vi "Burn-In Testing_v2.vi"() -> ()   [LabVIEW 2012]
uses:
  Controls/UserInput.ctl
  Controls/Instr_Param.ctl
  Controls/USB4000_Data.ctl
  Controls/MapPOS.ctl
  Controls/Waferimage.ctl
  Controls/MeasureControl.ctl
  Controls/TestArea.ctl
  Controls/TestData.ctl
  Controls/WaferTable.ctl
  Controls/Config.ctl
  Controls/AppPaths.ctl
  Controls/PathTraveler.ctl
  Controls/PathTypes.ctl
  Classes/EpiWrapper.lvclass
  TestData/Command.ctl
  Controls/Command_Enum.ctl
  Controls/Exit.vi
panel:
  in  "AppPaths":T1={"DataDir"={"Enum"=enum."DataDir", "FileName"="", "Exists?"=FALSE, "Path"=path ""}, "OmniDriver"={"Enum"=enum."OmniDriver", "FileName"="OmniDriver32.dll", "Exists?"=FALSE, "Path"=path ""}, "OmniDriverCommon"={"Enum"=enum."OmniDriver_Common", "FileName"="common32.dll", "Exists?"=FALSE, "Path"=path ""}, "Configuration"={"Enum"=enum."Configuration", "FileName"="TestConfiguration.cfg", "Exists?"=FALSE, "Path"=path ""}, "WaferImage"={"Enum"=enum."WaferImage", "FileName"="EPI_Wafer_Labels.jpg", "Exists?"=FALSE, "Path"=path ""}}
  in  "Configuration":T4={"IntTime"=100, "Samples"=3, "PowerMin"=300.0, "KneeMin"=-20.0, "KneeMax"=20.0, "BackgroundWl"=275.0} {"BackgroundWl" min=220.0 max=320.0; "IntTime" min=1 max=100000; "PowerMin" min=0.0 max=10000.0; "KneeMin" min=-40.0 max=0.0; "KneeMax" min=0.0 max=40.0; "Samples" min=1 max=10}
  out "Output For Excel":string
  in  "Integration Time(ms)\nMin=10ms":i32=10 min=10 max=100000
  out "Status":bool
  in  "Wafer Data,20mA":T5
  in  "MeasureControl":T6 {"TestData"."50mA Data"."Current,mA" format="%_6g"; "TestData"."50mA Data"."WL" format="%_6g"; "TestData"."50mA Data"."Voltage" format="%_6g"; "TestData"."50mA Data"."Power" format="%_6g"; "TestData"."20mA Data"."Reverse" format="%#_3g"; "TestData"."20mA Data"."Current,mA" format="%_6g"; "TestData"."20mA Data"."Knee Current" format="%#_3g"; "TestData"."20mA Data"."WL" format="%_6g"; "TestData"."20mA Data"."Voltage" format="%_6g"; "TestData"."20mA Data"."Power" format="%_5g"}
  out "Wafer":T9
  in  "MapPOS":T10={"Top"={"left"=208, "top"=106, "right"=218, "bottom"=116}, "CenterC"={"left"=217, "top"=189, "right"=228, "bottom"=200}, "CenterB"={"left"=217, "top"=208, "right"=228, "bottom"=219}, "CenterA"={"left"=199, "top"=208, "right"=209, "bottom"=219}, "Left"={"left"=103, "top"=199, "right"=114, "bottom"=209}, "Right"={"left"=314, "top"=199, "right"=325, "bottom"=209}}
  in  "INSTR_PARAM":T11
  in  "Stop":bool
  in  "Input":T13={"Wafer ID"="", "Test"="Initial", "New"=FALSE, "Save"=FALSE, "Load"=FALSE, "Cancel"=FALSE}
  # "Current Result"
  # "Measure Control"
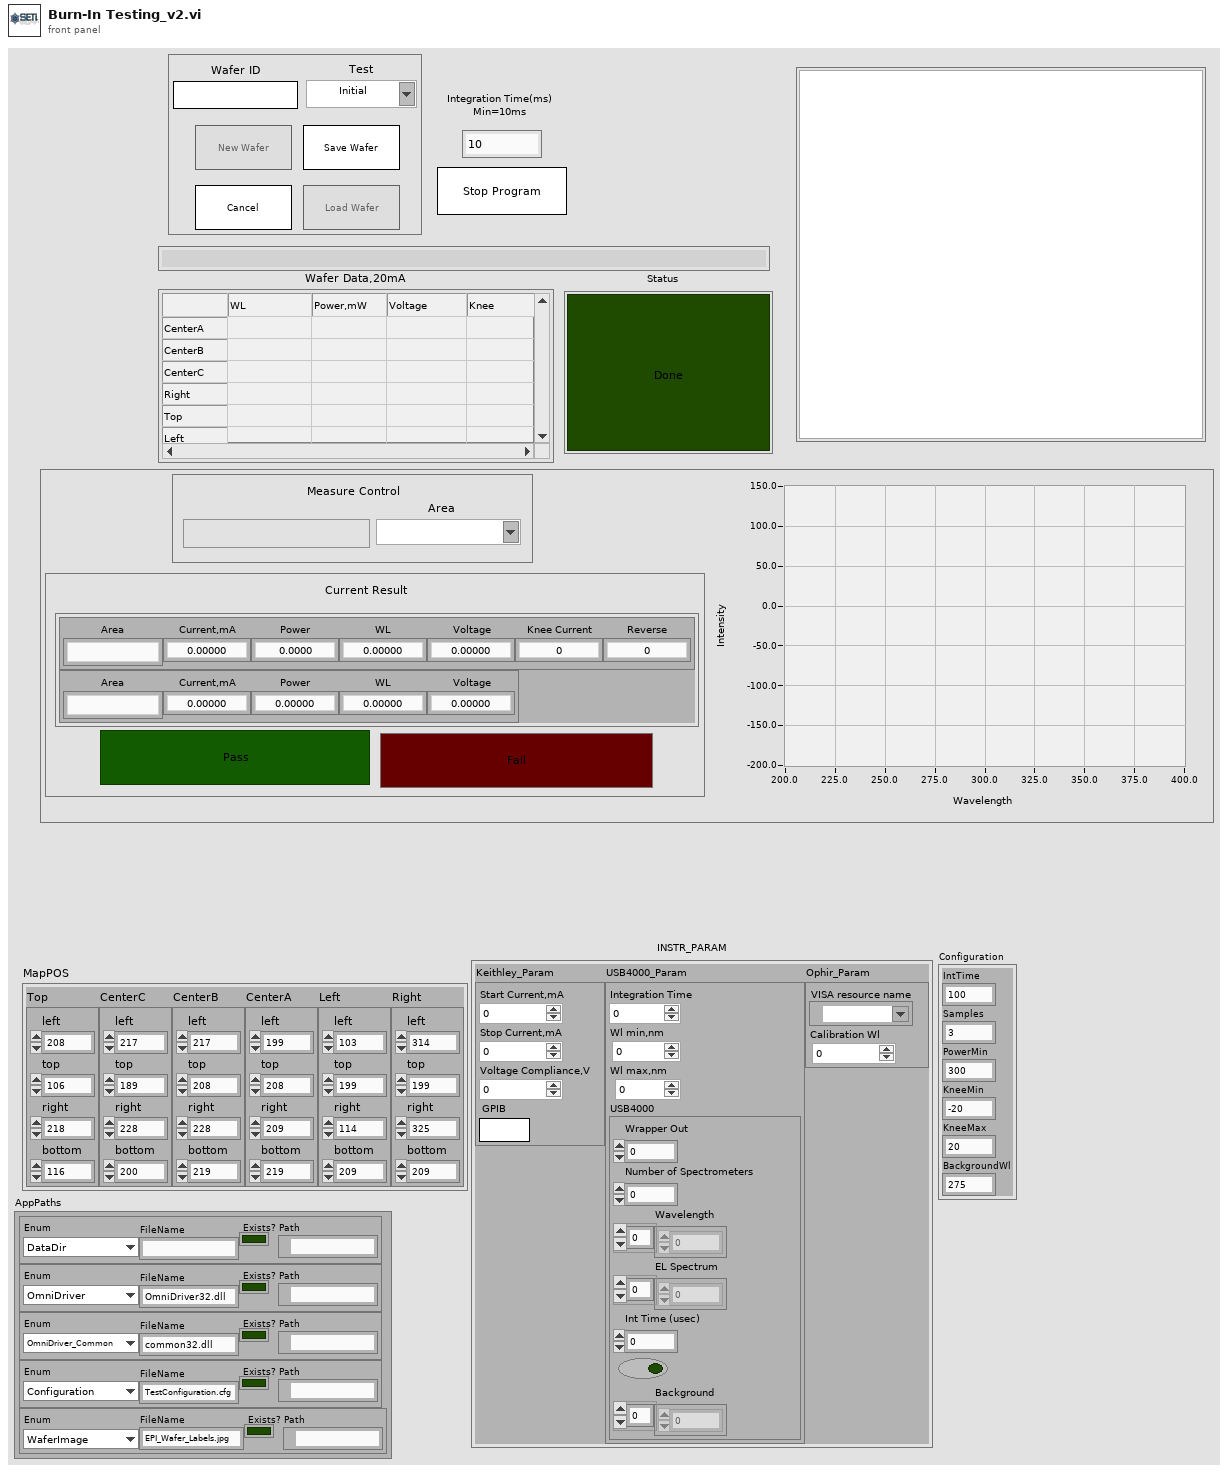
[diagram p1: front panel]
types:
  T1 = typedef "AppPaths.ctl" = cluster{"DataDir":T2, "OmniDriver":T2, "OmniDriverCommon":T2, "Configuration":T2, "WaferImage":T2}
  T2 = typedef "PathTraveler.ctl" = cluster{"Enum":T3, "FileName":string, "Exists?":bool, "Path":path}
  T3 = typedef "PathTypes.ctl" = enum16{"DataDir", "OmniDriver", "OmniDriver_Common", "Configuration", "WaferImage"}
  T4 = typedef "Config.ctl" = cluster{"IntTime":i32, "Samples":i32, "PowerMin":dbl, "KneeMin":dbl, "KneeMax":dbl, "BackgroundWl":dbl}
  T5 = typedef "WaferTable.ctl" = string[][]
  T6 = typedef "MeasureControl.ctl" = cluster{"Pass":bool, "Fail":bool, "Measure":bool, "Area":T7, "TestData":T8, "Graph":cluster{"Y":dbl[], "Y":dbl[]}[]}
  T7 = typedef "TestArea.ctl" = string
  T8 = typedef "TestData.ctl" = cluster{"20mA Data":cluster{"Area":string, "Current,mA":dbl, "Power":dbl, "WL":dbl, "Voltage":dbl, "Knee Current":dbl, "Reverse":dbl}, "50mA Data":cluster{"Area":string, "Current,mA":dbl, "Power":dbl, "WL":dbl, "Voltage":dbl}}
  T9 = typedef "Waferimage.ctl" = picture
  T10 = typedef "MapPOS.ctl" = cluster{"Top":cluster{"left":i16, "top":i16, "right":i16, "bottom":i16}, "CenterC":cluster{"left":i16, "top":i16, "right":i16, "bottom":i16}, "CenterB":cluster{"left":i16, "top":i16, "right":i16, "bottom":i16}, "CenterA":cluster{"left":i16, "top":i16, "right":i16, "bottom":i16}, "Left":cluster{"left":i16, "top":i16, "right":i16, "bottom":i16}, "Right":cluster{"left":i16, "top":i16, "right":i16, "bottom":i16}}
  T11 = typedef "Instr_Param.ctl" = cluster{"Keithley_Param":cluster{"Start Current,mA":dbl, "Stop Current,mA":dbl, "Voltage Compliance,V":dbl, "GPIB":string}, "USB4000_Param":cluster{"Integration Time":i32, "Wl min,nm":dbl, "Wl max,nm":dbl, "USB4000":T12}, "Ophir_Param":cluster{"VISA resource name":refnum<visa-resource-name>, "Calibration Wl":dbl}}
  T12 = typedef "USB4000_Data.ctl" = cluster{"Wrapper Out":u32, "Number of Spectrometers":i32, "Wavelength":dbl[], "EL Spectrum":dbl[], "Int Time (usec)":i32, bool, "Background":dbl[]}
  T13 = typedef "UserInput.ctl" = cluster{"Wafer ID":string, "Test":string, "New":bool, "Save":bool, "Load":bool, "Cancel":bool}
  T14 = typedef "Command.ctl" = cluster{"Command":T15, "Data":variant, "type":variant}
  T15 = typedef "Command_Enum.ctl" = enum16{"SPECTRUMCAPTURE", "RESETCONFIG", "OPENCONFIG", "RESET", "INIT", "LOAD", "MEASURE", "NEW", "SAVE", "UPDATE_INT", "SWAP_MODE", "UPDATE_ACQ", "EXIT", "CANCEL"}
  T16 = enum8{"Enabled", "Disabled", "Disabled and Grayed Out"}
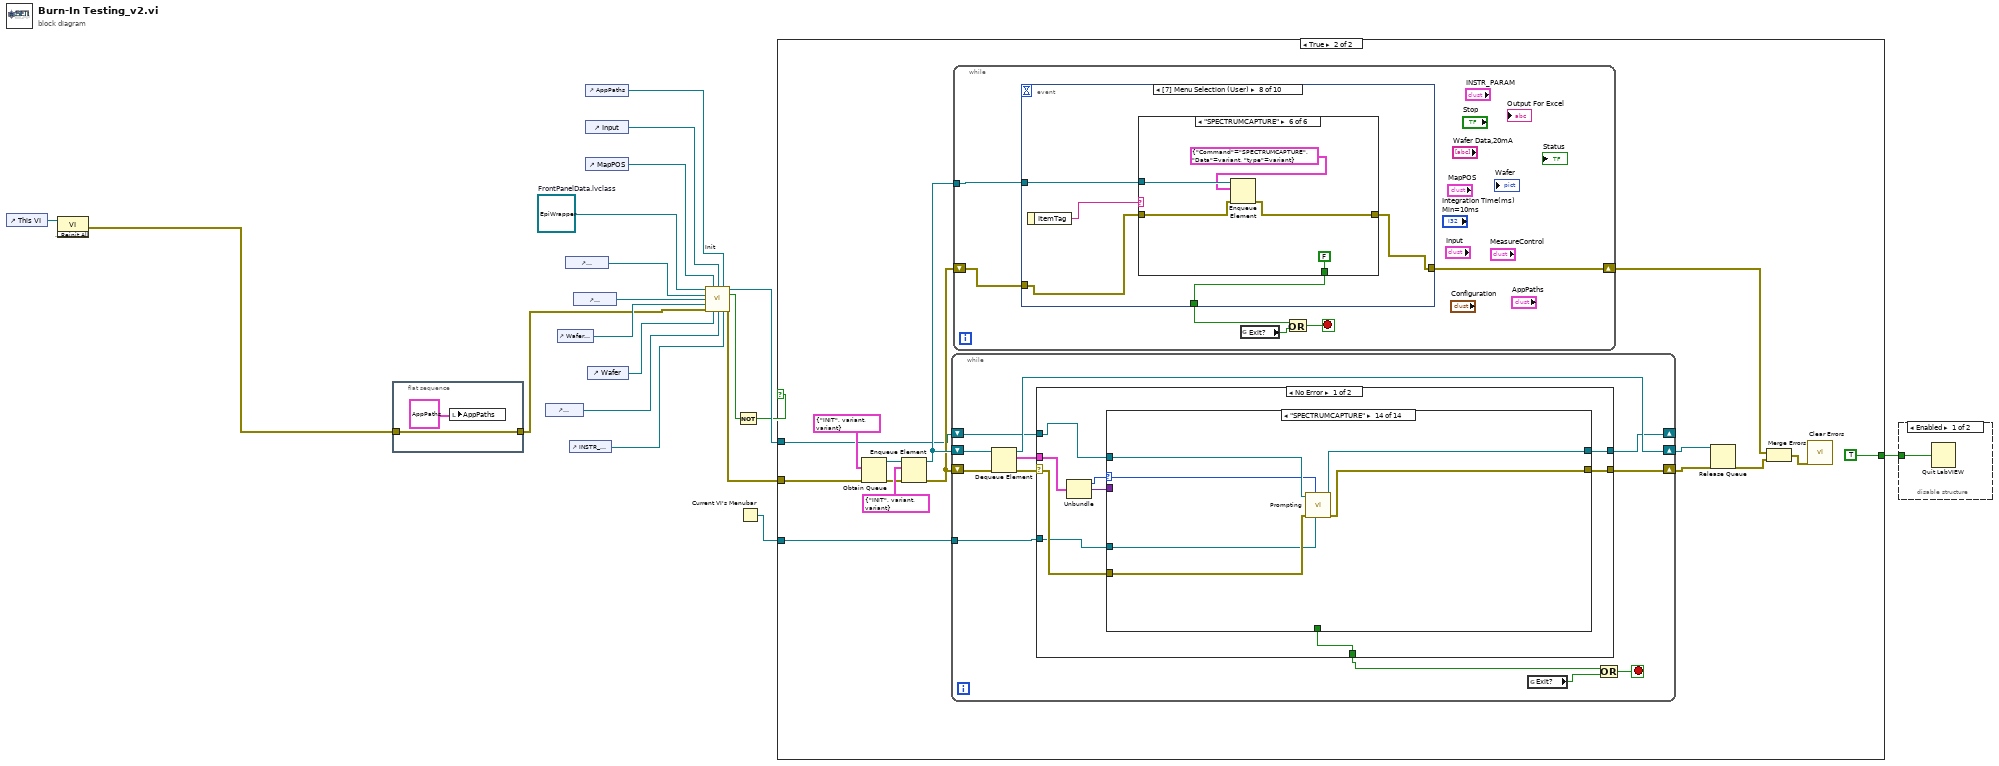
[diagram p0: block diagram]
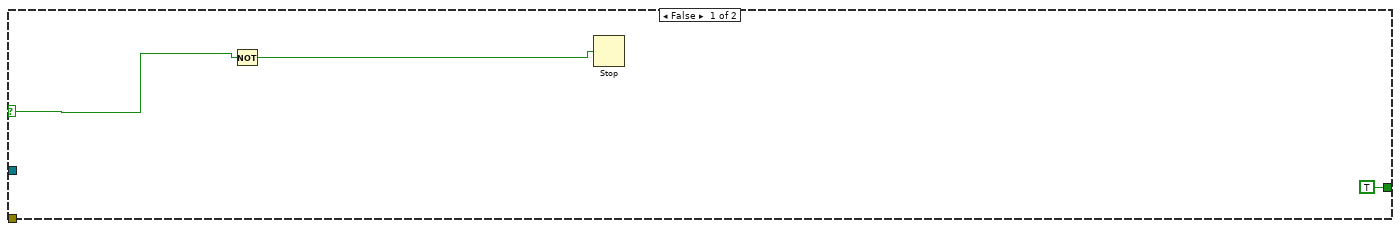
[diagram p3: hidden frame]
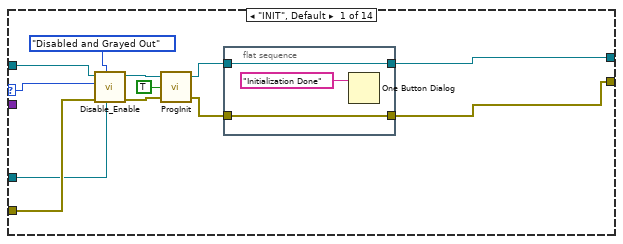
[diagram p4: hidden frame]
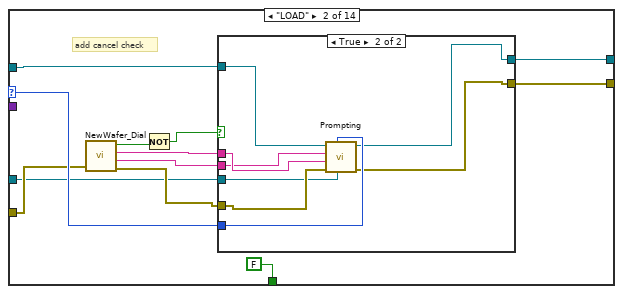
[diagram p5: hidden frame]
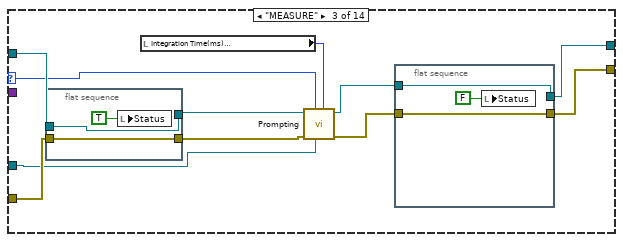
[diagram p7: hidden frame]
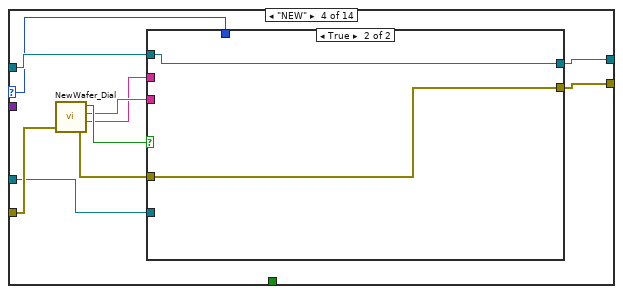
[diagram p8: hidden frame]
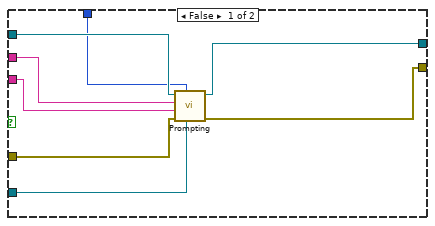
[diagram p9: hidden frame]
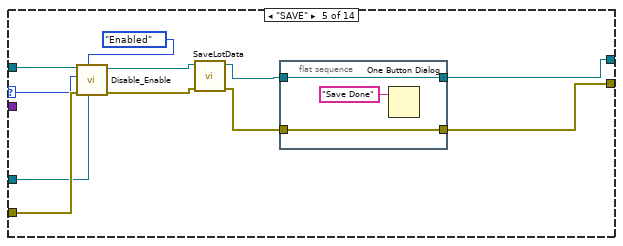
[diagram p10: hidden frame]
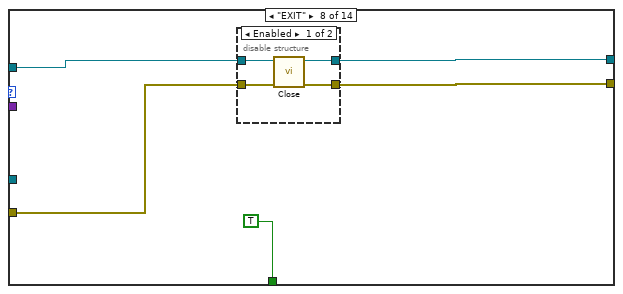
[diagram p13: hidden frame]
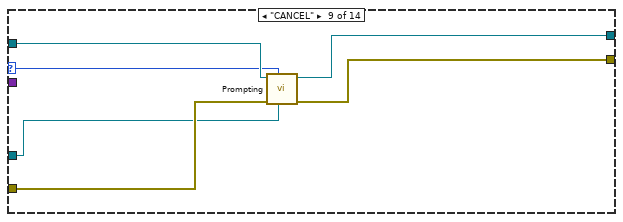
[diagram p15: hidden frame]
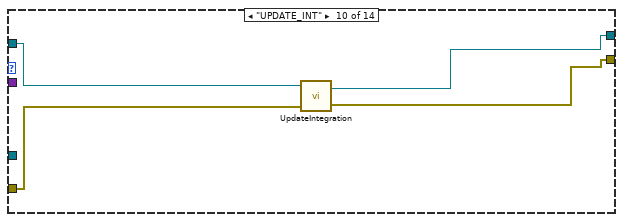
[diagram p16: hidden frame]
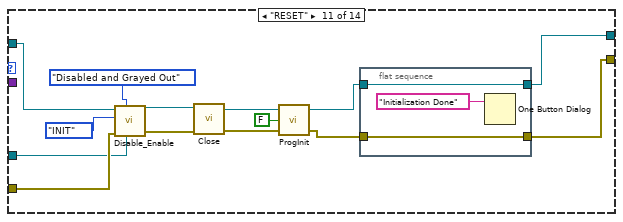
[diagram p17: hidden frame]
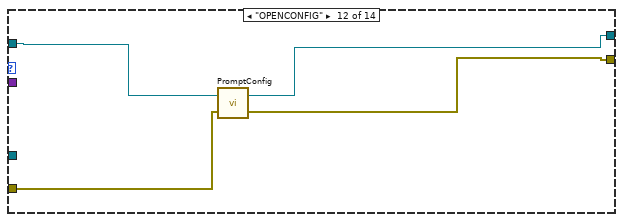
[diagram p18: hidden frame]
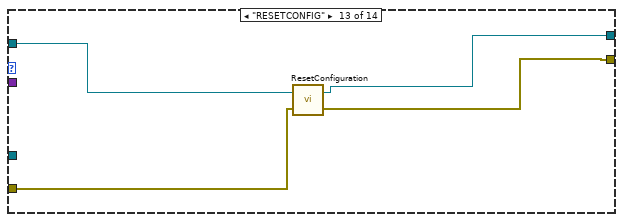
[diagram p19: hidden frame]
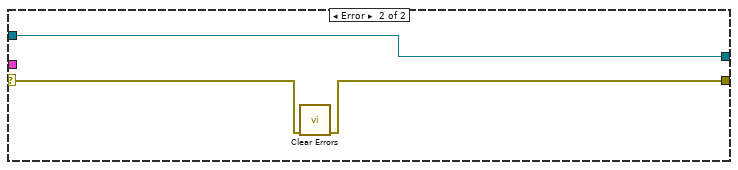
[diagram p20: hidden frame]
diagram:
  w19 = refnum<class "EpiWrapper.lvclass"> refnum  # FrontPanelData.lvclass
  n1 = control-ref of="This VI"() -> (w16:refnum<vi>)
  n2 = invoke class="VI" method="Default Vals.Reinit All"(reference=w16) -> (error out=w6:errorcluster)  [unwired: 2 in, 2 out]
  n3 = flat-sequence {
    tunnel: w6 -> [w21]
    tunnel: [w21] -> w5
    frame #0 {
      n4 = local write "AppPaths"(T1 {"DataDir"={"Enum"=enum."DataDir", "FileName"="", "Exists?"=FALSE, "Path"=path ""}, "OmniDriver"={"Enum"=enum."OmniDriver", "FileName"="OmniDriver32.dll", "Exists?"=FALSE, "Path"=path ""}, "OmniDriverCommon"={"Enum"=enum."OmniDriver_Common", "FileName"="common32.dll", "Exists?"=FALSE, "Path"=path ""}, "Configuration"={"Enum"=enum."Configuration", "FileName"="TestConfiguration.cfg", "Exists?"=FALSE, "Path"=path ""}, "WaferImage"={"Enum"=enum."WaferImage", "FileName"="EPI_Wafer_Labels.jpg", "Exists?"=FALSE, "Path"=path ""}} ("AppPaths")) -> ()
    }
  }
  n5 = control-ref of="Integration Time(ms)\nMin=10ms"() -> (w7:refnum<vi>)
  n6 = control-ref of="Wafer Data,20mA"() -> (w12:refnum<vi>)
  n7 = control-ref of="MeasureControl"() -> (w13:refnum<vi>)
  n8 = control-ref of="INSTR_PARAM"() -> (w10:refnum<vi>)
  n9 = control-ref of="Configuration"() -> (w4:refnum<vi>)
  n10 = control-ref of="AppPaths"() -> (w3:refnum<vi>)
  n11 = control-ref of="Input"() -> (w15:refnum<vi>)
  n12 = control-ref of="MapPOS"() -> (w14:refnum<vi>)
  n13 = control-ref of="Wafer"() -> (w11:refnum<vi>)
  n14 = call-dynamic "Init.vi"("FrontPanelData in"=w19, "MapPOS"=w14, "Input"=w15, "AppPaths"=w3, "MeasureControl"=w13, "Configuration"=w4, "WaferTablle_Ref"=w12, "error in (no error)"=w5, "Wafer"=w11, "IntTime_Ref"=w7, "INSTR_PARAM"=w10) -> ("FrontPanelData out"=w18:refnum<class "EpiWrapper.lvclass">, "Shutdown?"=w9:bool, "error out"=w17:errorcluster)  [unwired: 2 in]
  n15 = Not(x=w9) -> (.not. x?=w8:bool)
  n16 = Current VI's Menubar() -> (w1:refnum<k9>)
  n17 = case shown="True" w8 {
    selector: w8 -> [w23 _]
    tunnel: w18 -> [_ w34]
    tunnel: w17 -> [_ w33]
    tunnel: [TRUE ("quit? (T)") TRUE ("quit? (T)")] -> w2
    tunnel: w1 -> [_ w25]
    frame False {
      n18 = Not(x=w23) -> (.not. x?=w22:bool)
      n19 = Stop(stop? (T)=w22) -> ()
    }
    frame True {
      n20 = Obtain Queue(element data type=T14 {"Command"=enum."INIT", "Data"=variant, "type"=variant} ("Cluster"), error in (no error)=w33) -> (queue out=w37:refnum<queue>, error out=w32:errorcluster)  [unwired: 3 in, 1 out]
      n21 = Enqueue Element(queue=w37, element=T14 {"Command"=enum."INIT", "Data"=variant, "type"=variant}, error in (no error)=w32) -> (queue out=w39:refnum<queue>, error out=w35:errorcluster)  [unwired: 1 in, 1 out]
      n22 = while {
        shift-right: [w47] -> w31
        shift-left: w39 -> [w51]
        shift-right: [w48] -> w30
        shift-left: w35 -> [w49]
        shift-right: [w41] -> _
        shift-left: w34 -> [w42]
        tunnel: w25 -> [w40]
        stop <- w44 stop-if-true
        n23 = Dequeue Element(queue=w51, error in (no error)=w49) -> (queue out=w47:refnum<queue>, element=w46:T14, error out=w50:errorcluster)  [unwired: 1 in, 1 out]
        n24 = case shown="No Error" w50 {
          selector: w50 -> [w56 w206]
          tunnel: [w57 w205] -> w48
          tunnel: w46 -> [w60 _]
          tunnel: [w58 _] -> w43
          tunnel: w42 -> [w55 w207]
          tunnel: [w54 w207] -> w41
          tunnel: w40 -> [w52 _]
          frame No Error {
            n25 = Unbundle(w60) -> ("Command"=w59:T15, "Data"=w53:variant)  [unwired: 1 out]
            n26 = case shown="\"SPECTRUMCAPTURE\"" w59 {
              selector: w59 -> [w65 w81 w101 w118 w136 _ _ _ w165 _ _ _ _ w200]
              tunnel: [_ FALSE ("y") _ _ _ _ _ TRUE ("y") _ _ _ _ _ _] -> w58
              tunnel: [w63 w82 w98 w119 w138 w150 w152 w153 w167 w170 w177 w193 w196 w202] -> w57
              tunnel: w56 -> [w69 w78 w107 w117 w144 w150 w152 w155 w168 w172 w185 w191 w197 w203]
              tunnel: w55 -> [w70 w84 w108 w121 w145 w149 w151 w156 w169 w173 w186 w194 w198 w204]
              tunnel: [w64 w83 w104 w120 w137 w149 w151 w154 w166 w171 w176 w192 w195 w201] -> w54
              tunnel: w53 -> [_ _ _ _ _ _ _ _ _ _ _ _ _ _]
              tunnel: w52 -> [w62 w76 w99 w115 w135 _ _ _ w164 _ w175 _ _ w199]
              frame "INIT", Default {
                n27 = call-dynamic "Disable_Enable.vi"("menu reference"=w62, "Disabled"=T16."Disabled and Grayed Out", "error in (no error)"=w69, "Command"=w65, "EpiWrapper in"=w70) -> ("error out"=w67:errorcluster, "EpiWrapper out"=w68:refnum<class "EpiWrapper.lvclass">)  [unwired: 5 in]
                n28 = call-dynamic "ProgInit.vi"("error in (no error)"=w67, "Intialize?"=TRUE, "EpiWrapper in"=w68) -> ("error out"=w72:errorcluster, "EpiWrapper out"=w71:refnum<class "EpiWrapper.lvclass">)  [unwired: 1 in]
                n29 = flat-sequence {
                  tunnel: [w74] -> w63
                  tunnel: w72 -> [w74]
                  tunnel: [w73] -> w64
                  tunnel: w71 -> [w73]
                  frame #0 {
                    n30 = One Button Dialog(message="Initialization Done") -> ()  [unwired: 1 in, 1 out]
                  }
                }
              }
              frame "LOAD" {
                # "add cancel check"
                n31 = call "NewWafer_Dial.vi"("error in (no error)"=w78) -> ("Cancelled?"=w80:bool, "Test Out"=w85:string, "Wafer ID Out"=w86:string, "error out"=w77:errorcluster)  [unwired: 2 in]
                n32 = Not(x=w80) -> (.not. x?=w79:bool)
                n33 = case shown="True" w79 {
                  tunnel: w86 -> [_ w93]
                  tunnel: w85 -> [_ w94]
                  tunnel: w77 -> [w88 w95]
                  tunnel: w84 -> [w89 w97]
                  tunnel: [w89 w92] -> w83
                  tunnel: [w88 w91] -> w82
                  tunnel: w81 -> [_ w96]
                  tunnel: w76 -> [_ w90]
                  frame False {
                  }
                  frame True {
                    n34 = call-dynamic "Prompting.vi"("menu reference"=w90, "Command"=w96, "error in (no error)"=w95, "Type"=w94, "Wafer ID"=w93, "EpiWrapper in"=w97) -> ("error out"=w91:errorcluster, "EpiWrapper out"=w92:refnum<class "EpiWrapper.lvclass">)  [unwired: 4 in]
                  }
                }
              }
              frame "MEASURE" {
                n35 = flat-sequence {
                  tunnel: [w113] -> w106
                  tunnel: w108 -> [w113]
                  tunnel: w107 -> [w112]
                  tunnel: [w112] -> w100
                  frame #0 {
                    n36 = local write "Status"(TRUE ("Status")) -> ()
                  }
                }
                n37 = local read "Integration Time(ms)\nMin=10ms"() -> (w102:i32)
                n38 = call-dynamic "Prompting.vi"("New Integration Time"=w102, "menu reference"=w99, "Command"=w101, "error in (no error)"=w100, "EpiWrapper in"=w106) -> ("error out"=w105:errorcluster, "EpiWrapper out"=w103:refnum<class "EpiWrapper.lvclass">)  [unwired: 5 in]
                n39 = flat-sequence {
                  tunnel: w105 -> [w109]
                  tunnel: [w110] -> w104
                  tunnel: w103 -> [w110]
                  tunnel: [w109] -> w98
                  frame #0 {
                    n40 = local write "Status"(FALSE ("Status")) -> ()
                  }
                }
              }
              frame "NEW" {
                n41 = call "NewWafer_Dial.vi"("error in (no error)"=w117) -> ("Cancelled?"=w124:bool, "Test Out"=w123:string, "Wafer ID Out"=w122:string, "error out"=w116:errorcluster)  [unwired: 2 in]
                n42 = case shown="True" w124 {
                  tunnel: w123 -> [w127 _]
                  tunnel: w122 -> [w128 _]
                  tunnel: w121 -> [w132 w134]
                  tunnel: w116 -> [w131 w133]
                  tunnel: [w130 w134] -> w120
                  tunnel: [w129 w133] -> w119
                  tunnel: w118 -> [w126 _]
                  tunnel: w115 -> [w125 _]
                  frame False {
                    n43 = call-dynamic "Prompting.vi"("menu reference"=w125, "Command"=w126, "error in (no error)"=w131, "Type"=w127, "Wafer ID"=w128, "EpiWrapper in"=w132) -> ("error out"=w129:errorcluster, "EpiWrapper out"=w130:refnum<class "EpiWrapper.lvclass">)  [unwired: 4 in]
                  }
                  frame True {
                  }
                }
              }
              frame "SAVE" {
                n44 = call-dynamic "Disable_Enable.vi"("menu reference"=w135, "Disabled"=T16."Enabled", "error in (no error)"=w144, "Command"=w136, "EpiWrapper in"=w145) -> ("error out"=w141:errorcluster, "EpiWrapper out"=w142:refnum<class "EpiWrapper.lvclass">)  [unwired: 5 in]
                n45 = call-dynamic "SaveLotData.vi"("error in (no error)"=w141, "EpiWrapper in"=w142) -> ("error out"=w139:errorcluster, "EpiWrapper out"=w140:refnum<class "EpiWrapper.lvclass">)  [unwired: 8 in]
                n46 = flat-sequence {
                  tunnel: [w147] -> w138
                  tunnel: w139 -> [w147]
                  tunnel: [w146] -> w137
                  tunnel: w140 -> [w146]
                  frame #0 {
                    n47 = One Button Dialog(message="Save Done") -> ()  [unwired: 1 in, 1 out]
                  }
                }
              }
              frame "SWAP_MODE" {
              }
              frame "UPDATE_ACQ" {
              }
              frame "EXIT" {
                n48 = disable-structure shown="Enabled" {
                  disable-tunnel: w156 -> [w161 w163]
                  disable-tunnel: w155 -> [w160 w162]
                  disable-tunnel: [w159 w163] -> w154
                  disable-tunnel: [w158 w162] -> w153
                  frame Enabled {
                    n49 = call-dynamic "Close.vi"("error in (no error)"=w160, "EpiWrapper in"=w161) -> ("error out"=w158:errorcluster, "EpiWrapper out"=w159:refnum<class "EpiWrapper.lvclass">)  [unwired: 8 in]
                  }
                  frame Disabled {
                  }
                }
              }
              frame "CANCEL" {
                n50 = call-dynamic "Prompting.vi"("menu reference"=w164, "Command"=w165, "error in (no error)"=w168, "EpiWrapper in"=w169) -> ("error out"=w167:errorcluster, "EpiWrapper out"=w166:refnum<class "EpiWrapper.lvclass">)  [unwired: 6 in]
              }
              frame "UPDATE_INT" {
                n51 = call-dynamic "UpdateIntegration.vi"("error in (no error)"=w172, "EpiWrapper in"=w173) -> ("error out"=w170:errorcluster, "EpiWrapper out"=w171:refnum<class "EpiWrapper.lvclass">)  [unwired: 1 in]
              }
              frame "RESET" {
                n52 = call-dynamic "Disable_Enable.vi"("menu reference"=w175, "Disabled"=T16."Disabled and Grayed Out", "error in (no error)"=w185, "Command"=Command_Enum."INIT", "EpiWrapper in"=w186) -> ("error out"=w182:errorcluster, "EpiWrapper out"=w183:refnum<class "EpiWrapper.lvclass">)  [unwired: 5 in]
                n53 = call-dynamic "Close.vi"("error in (no error)"=w182, "EpiWrapper in"=w183) -> ("error out"=w180:errorcluster, "EpiWrapper out"=w181:refnum<class "EpiWrapper.lvclass">)  [unwired: 8 in]
                n54 = call-dynamic "ProgInit.vi"("error in (no error)"=w180, "Intialize?"=FALSE, "EpiWrapper in"=w181) -> ("error out"=w178:errorcluster, "EpiWrapper out"=w179:refnum<class "EpiWrapper.lvclass">)  [unwired: 1 in]
                n55 = flat-sequence {
                  tunnel: [w189] -> w177
                  tunnel: w178 -> [w189]
                  tunnel: [w188] -> w176
                  tunnel: w179 -> [w188]
                  frame #0 {
                    n56 = One Button Dialog(message="Initialization Done") -> ()  [unwired: 1 in, 1 out]
                  }
                }
              }
              frame "OPENCONFIG" {
                n57 = call-dynamic "PromptConfig.vi"("error in (no error)"=w191, "EpiWrapper in"=w194) -> ("error out"=w193:errorcluster, "EpiWrapper out"=w192:refnum<class "EpiWrapper.lvclass">)
              }
              frame "RESETCONFIG" {
                n58 = call-dynamic "ResetConfiguration.vi"("error in (no error)"=w197, "EpiWrapper in"=w198) -> ("error out"=w196:errorcluster, "EpiWrapper out"=w195:refnum<class "EpiWrapper.lvclass">)
              }
              frame "SPECTRUMCAPTURE" {
                n59 = call-dynamic "Prompting.vi"("menu reference"=w199, "Command"=w200, "error in (no error)"=w203, "EpiWrapper in"=w204) -> ("error out"=w202:errorcluster, "EpiWrapper out"=w201:refnum<class "EpiWrapper.lvclass">)  [unwired: 6 in]
              }
            }
          }
          frame Error {
            n60 = call <vilib>:"Clear Errors.vi"("error in (no error)"=w206) -> ("error out"=w205:errorcluster)  [unwired: 6 in]
          }
        }
        n61 = global read "Exit.vi" "Exit?"() -> (w45:bool)
        n62 = Or(x=w43, y=w45) -> (x .or. y?=w44:bool)
      }
      n63 = while {
        tunnel: w39 -> [w213]
        shift-right: [w208] -> w27
        shift-left: w35 -> [w209]
        stop <- w211 stop-if-true
        n64 = event shown="[7] Menu Selection (User)" {
          selector: _ -> [_ _ _ _ _ _ _ _ _ _]
          dyn-events: _ -> [_ _ _ _ _ _ _ _ _ _]
          timeout: _ -> [_ _ _ _ _ _ _ _ _ _]
          tunnel: w213 -> [_ w218 w222 w227 w230 w234 w238 w243 w275 w279]
          tunnel: [_ TRUE ("x") _ _ _ _ _ w240 TRUE ("x") _] -> w210
          tunnel: w209 -> [w214 w216 w221 w226 w229 w233 w237 w242 w274 w278]
          tunnel: [w214 w215 w220 w224 w228 w235 w236 w241 w272 w277] -> w208
          event Timeout {
            n65 = event-data() -> ()  [unwired: 1 in, 2 out]
          }
          event "Stop": Value Change {
            n66 = event-data() -> ()  [unwired: 1 in, 5 out]
            n67 = Enqueue Element(queue=w218, element=T14 {"Command"=enum."EXIT", "Data"=variant, "type"=variant}, error in (no error)=w216) -> (error out=w215:errorcluster)  [unwired: 1 in, 2 out]
          }
          event Value Change {
            n68 = event-data() -> ()  [unwired: 1 in, 5 out]
            n69 = Enqueue Element(queue=w222, element=T14 {"Command"=enum."SAVE", "Data"=variant, "type"=variant}, error in (no error)=w221) -> (error out=w220:errorcluster)  [unwired: 1 in, 2 out]
          }
          event Value Change {
            n70 = event-data() -> ()  [unwired: 1 in, 5 out]
            n71 = Enqueue Element(queue=w227, element=T14 {"Command"=enum."MEASURE", "Data"=variant, "type"=variant}, error in (no error)=w226) -> (error out=w224:errorcluster)  [unwired: 1 in, 2 out]
          }
          event Value Change {
            n72 = event-data() -> ()  [unwired: 1 in, 5 out]
            n73 = Enqueue Element(queue=w230, element=T14 {"Command"=enum."CANCEL", "Data"=variant, "type"=variant}, error in (no error)=w229) -> (error out=w228:errorcluster)  [unwired: 1 in, 2 out]
          }
          event Value Change {
            n74 = event-data() -> ()  [unwired: 1 in, 5 out]
            n75 = Enqueue Element(queue=w234, element=T14 {"Command"=enum."NEW", "Data"=variant, "type"=variant}, error in (no error)=w233) -> (error out=w235:errorcluster)  [unwired: 1 in, 2 out]
          }
          event Value Change {
            n76 = event-data() -> ()  [unwired: 1 in, 5 out]
            n77 = Enqueue Element(queue=w238, element=T14 {"Command"=enum."LOAD", "Data"=variant, "type"=variant}, error in (no error)=w237) -> (error out=w236:errorcluster)  [unwired: 1 in, 2 out]
          }
          event Menu Selection (User) {
            n78 = event-data() -> ("ItemTag"=w244:string)  [unwired: 1 in]
            n79 = case shown="\"SPECTRUMCAPTURE\"" w244 {
              tunnel: w243 -> [_ w250 w253 w260 w265 w271]
              tunnel: w242 -> [w246 w249 w254 w259 w264 w269]
              tunnel: [w246 w248 w255 w258 w263 w268] -> w241
              tunnel: [FALSE ("x") FALSE ("x") TRUE ("x") FALSE ("x") FALSE ("x") FALSE ("x")] -> w240
              frame "False", Default {
              }
              frame "OPENCONFIG" {
                n80 = Enqueue Element(queue=w250, element=T14 {"Command"=enum."OPENCONFIG", "Data"=variant, "type"=variant}, error in (no error)=w249) -> (error out=w248:errorcluster)  [unwired: 1 in, 2 out]
              }
              frame "EXIT" {
                n81 = Enqueue Element(queue=w253, element=T14 {"Command"=enum."EXIT", "Data"=variant, "type"=variant}, error in (no error)=w254) -> (error out=w255:errorcluster)  [unwired: 1 in, 2 out]
              }
              frame "RESET" {
                n82 = Enqueue Element(queue=w260, element=T14 {"Command"=enum."RESET", "Data"=variant, "type"=variant}, error in (no error)=w259) -> (error out=w258:errorcluster)  [unwired: 1 in, 2 out]
              }
              frame "RESETCONFIG" {
                n83 = Enqueue Element(queue=w265, element=T14 {"Command"=enum."RESETCONFIG", "Data"=variant, "type"=variant}, error in (no error)=w264) -> (error out=w263:errorcluster)  [unwired: 1 in, 2 out]
              }
              frame "SPECTRUMCAPTURE" {
                n84 = Enqueue Element(queue=w271, element=T14 {"Command"=enum."SPECTRUMCAPTURE", "Data"=variant, "type"=variant}, error in (no error)=w269) -> (error out=w268:errorcluster)  [unwired: 1 in, 2 out]
              }
            }
          }
          event Panel Close {
            n85 = event-data() -> ()  [unwired: 1 in, 4 out]
            n86 = Enqueue Element(queue=w275, element=T14 {"Command"=enum."EXIT", "Data"=variant, "type"=variant}, error in (no error)=w274) -> (error out=w272:errorcluster)  [unwired: 1 in, 2 out]
          }
          event "Integration Time(ms)\nMin=10ms": Value Change {
            n87 = event-data() -> ()  [unwired: 1 in, 5 out]
            n88 = Enqueue Element(queue=w279, element=T14 {"Command"=enum."UPDATE_INT", "Data"=variant, "type"=variant}, error in (no error)=w278) -> (error out=w277:errorcluster)  [unwired: 1 in, 2 out]
          }
        }
        n89 = global read "Exit.vi" "Exit?"() -> (w212:bool)
        n90 = Or(x=w210, y=w212) -> (x .or. y?=w211:bool)
      }
      n91 = Release Queue(queue=w31, error in (no error)=w30) -> (error out=w29:errorcluster)  [unwired: 1 in, 2 out]
      n92 = Merge Errors(w27, w29) -> (w28:errorcluster)
      n93 = call <vilib>:"Clear Errors.vi"("error in (no error)"=w28) -> ()  [unwired: 6 in, 1 out]
    }
  }
  n94 = disable-structure shown="Enabled" {
    disable-tunnel: w2 -> [w281 _]
    frame Enabled {
      n95 = Quit LabVIEW(quit? (T)=w281) -> ()
    }
    frame Disabled {
    }
  }
